vi "StageInitialize.vi"(8 "error in (no error)":errorcluster, 9 "HWSerialNum":i32=94839332, 10 "MG17Motor In":refnum<k7>, 11 "Microscope in":refnum<class "Microscope.lvclass">) -> (0 "error out":errorcluster, 2 "MG17Motor Out":refnum<k7>, 3 "Microscope out":refnum<class "Microscope.lvclass">)   [LabVIEW 2012, in "Microscope.lvclass"]
uses:
  classes/Microscope.lvclass
  classes/Microscope.lvclass/Microscope.ctl
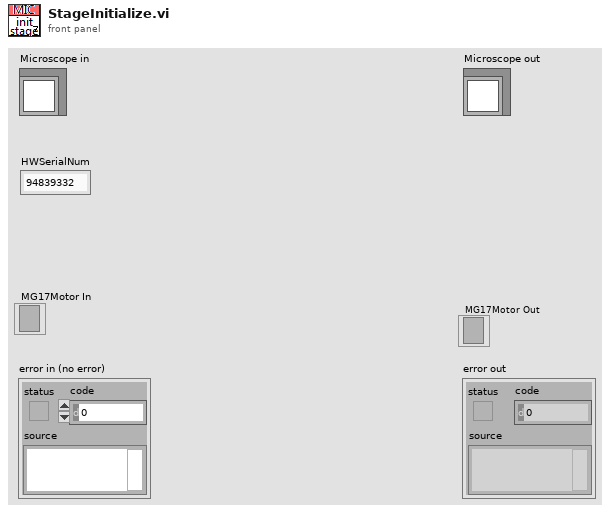
[diagram p1: front panel]
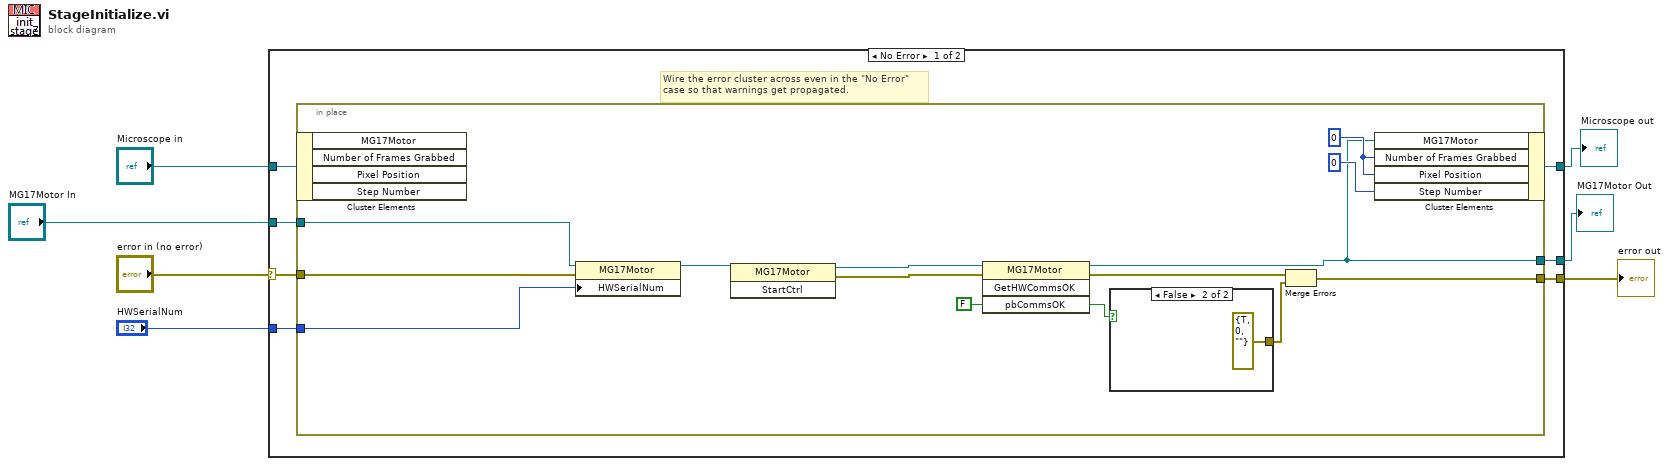
[diagram p0: block diagram]
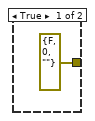
[diagram p2: hidden frame]
diagram:
  n1 = case shown="No Error" "error in (no error)" {
    selector: "error in (no error)" -> [w10 w32]
    tunnel: [w9 w32] -> w6
    tunnel: [w12 w31] -> w4
    tunnel: "Microscope in" -> [w13 w31]
    tunnel: "HWSerialNum" -> [w14 _]
    tunnel: [w11 _] -> w2
    tunnel: "MG17Motor In" -> [w8 _]
    frame No Error {
      # "Wire the error cluster across even in the \"No Error\"\ncase so that warnings get propagated."
      n2 = in-place {
        in-place-border: w14 -> [w28]
        in-place-border: [w25] -> w11
        in-place-border: w10 -> [w17]
        in-place-border: [w24] -> w9
        in-place-border: w8 -> [w15]
        w26 = 0 ("Pixel Position")
        n3 = in-place-cluster #1(w13) -> ()  [unwired: 4 out]
        n4 = property class="MG17Motor"(reference=w15, error in=w17, "HWSerialNum"=w28) -> (reference out=w18:refnum<k7>)  [unwired: 1 out]
        n5 = invoke class="MG17Motor" method="StartCtrl"(reference=w18) -> (reference out=w20:refnum<k7>, error out=w19:errorcluster)  [unwired: 2 in, 1 out]
        n6 = invoke class="MG17Motor" method="GetHWCommsOK"(reference=w20, error in=w19, "pbCommsOK"=FALSE) -> (reference out=w25:refnum<k7>, error out=w22:errorcluster, "pbCommsOK"=w23:bool)  [unwired: 1 in, 1 out]
        n7 = case shown="False" w23 {
          tunnel: [errorcluster {"status"=FALSE, "code"=0, "source"=""} ("error in (no error)") errorcluster {"status"=TRUE, "code"=0, "source"=""} ("error in (no error)")] -> w21
          frame True {
          }
          frame False {
          }
        }
        n8 = Merge Errors(w22, w21) -> (w24:errorcluster)
        n9 = in-place-cluster #1("MG17Motor"=w25, "Number of Frames Grabbed"=w26, "Pixel Position"=w26, "Step Number"=0 ("Stage Acquire Parameters.step number")) -> (w12:refnum<class "Microscope.lvclass">)
      }
    }
    frame Error {
    }
  }
  "error out" <- w6
  "Microscope out" <- w4
  "MG17Motor Out" <- w2
